vi "已用时间定时器（时钟).vi"(7 "Elapsed Time Target":dbl=12.0 caption="目标所需时间" format="%0.8f", 8 "error in (no error)":errorcluster caption="错误输入（无错误）", 9 "Auto Reset":bool=TRUE caption="自动重置", 10 "设置起始时间":timestamp, 11 "Reset":bool caption="重置") -> (0 "error out":errorcluster caption="错误输出", 2 "Elapsed Time":dbl caption="已用时间" format="%0.2f", 3 "Time has Elapsed":bool caption="结束")   [LabVIEW 2012]
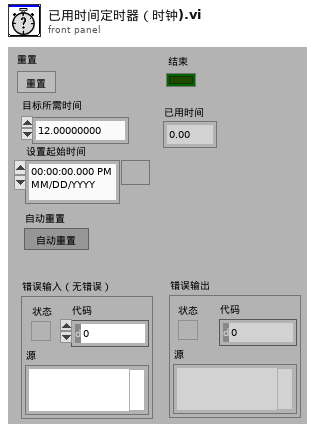
[diagram p1: front panel]
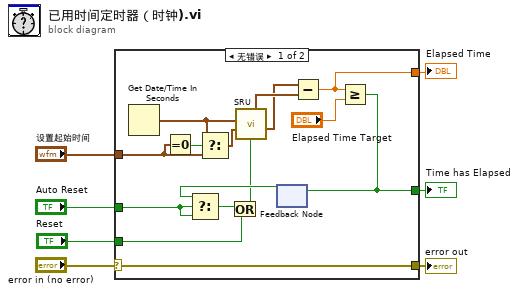
[diagram p0: block diagram]
diagram:
  n1 = case shown="无错误" "error in (no error)" {
    selector: "error in (no error)" -> [w17 w23]
    tunnel: [w17 w23] -> w6
    tunnel: "设置起始时间" -> [w11 _]
    tunnel: "Auto Reset" -> [w16 _]
    tunnel: "Reset" -> [w15 _]
    tunnel: [w14 _] -> w2
    tunnel: [w13 _] -> w1
    frame No Error {
      n2 = Get Date/Time In Seconds() -> (seconds since 1Jan1904=w9:timestamp)
      n3 = Equal To 0?(x=w11) -> (x = 0?=w12:bool)
      n4 = Select(t=w9, s=w12, f=w11) -> (s? t:f=w10:timestamp)
      n5 = feedback #1() -> (w20:bool)  [unwired: 1 in]
      n6 = Select(t=w20, s=w16, f=w16) -> (s? t:f=w19:bool)
      n7 = Or(x=w19, y=w15) -> (x .or. y?=w18:bool)
      n8 = call-poly "SRU.vi"("复位"=w18, "初始值"=w10, "输入"=w9) -> ("本次值"=w8:timestamp, "初始值"=w21:timestamp)  [unwired: 6 in, 1 out]
      n9 = Subtract(x=w8, y=w21) -> (x-y=w13:dbl)
      n10 = Greater Or Equal?(x=w13, y="Elapsed Time Target") -> (x >= y?=w14:bool)
      n11 = feedback-in #1(w14) -> ()
    }
    frame Error {
    }
  }
  "error out" <- w6
  "Time has Elapsed" <- w2
  "Elapsed Time" <- w1
